vi "host.vi"() -> ()   [LabVIEW 2020]
uses:
  b4957acc-33c7-4f51-b6c8-be02e890b770.vi
  <vilib>/Array/Sort 2D Array - Pop Stack.vi
  <vilib>/Array/Sort 2D Array - Push Stack.vi
  b4957acc-33c7-4f51-b6c8-be02e890b770.vi/269d4b3b-47f5-49e3-8884-44851e4dd9d5.vi
  b4957acc-33c7-4f51-b6c8-be02e890b770.vi/6d99389c-673d-4efb-bf33-19b32bcf4cf8.vi
  <vilib>/FPGAPlugInAG/cRIO-9054/niLvFpga_Open_cRIO-9054.vi
  <vilib>/FPGAPlugInAG/cRIO-9054/niLvFpga_Reset_cRIO-9054.vi
  <vilib>/Utility/error.llb/Error Cluster From Error Code.vi
  <vilib>/rvi/errors/niLvFpgaAdjustHostInterfaceError.vi
  <vilib>/FPGAPlugInAG/cRIO-9054/niLvFpga_Run_cRIO-9054.vi
  <vilib>/FPGAPlugInAG/cRIO-9054/niLvFpga_Close_cRIO-9054.vi
  <vilib>/rvi/interface/nirviOpenFPGA/nirviOpenFPGA.xnode
  FPGA Bitfiles/latchproject_FPGATarget_FPGALatch2_iIOhPE-h5cE.lvbitx
  <vilib>/rvi/interface/nirviMethod/nirviMethod.xnode
  <vilib>/rvi/interface/nirviReadWriteControl/nirviReadWriteControl.xnode
  <vilib>/rvi/interface/nirviCloseFPGA/nirviCloseFPGA.xnode
  <vilib>/Analysis/NI_AALBase.lvlib
  <vilib>/rvi/errors/niLvFpgaMergeErrorWithErrorCode.vi
  <vilib>/FPGAPlugInAG/cRIO-9054/niLvFpga_StartFifo_cRIO-9054.vi
  <vilib>/FPGAPlugInAG/cRIO-9054/niLvFpga_ReadFifo_cRIO-9054.vi
  <vilib>/FPGAPlugInAG/cRIO-9054/niLvFpga_WriteFifo_cRIO-9054.vi
  NiFpgaLv.dll
panel:
  out "Timed Out? FIFO out index":bool
  out "Timed Out? FIFO out IMG":bool
  out "Timed Out? FIFO out REAL":bool
  out "Timed Out? FIFO in REAL":bool
  out "Timed Out? FIFO in IMG":bool
  out "sorted signal 3":dbl[](graph)
  out "Data":fxp<+/-,32,21>[](array[numeric])
  out "sorted signal 2":dbl[](graph)
  out "index values":i32[](array[numeric])
  out "sorted 2D array":dbl[][](array[numeric])
  out "appended array":dbl[][](array[numeric])
  out "sorted array":dbl[](array[numeric])
  out "uniform white noise":dbl[](array[numeric])
  out "Waveform Graph":sgl[](graph)
  out "sort time (ms)":dbl
  out "Elements Remaining":u32
  out "sorted signal":dbl[](graph)
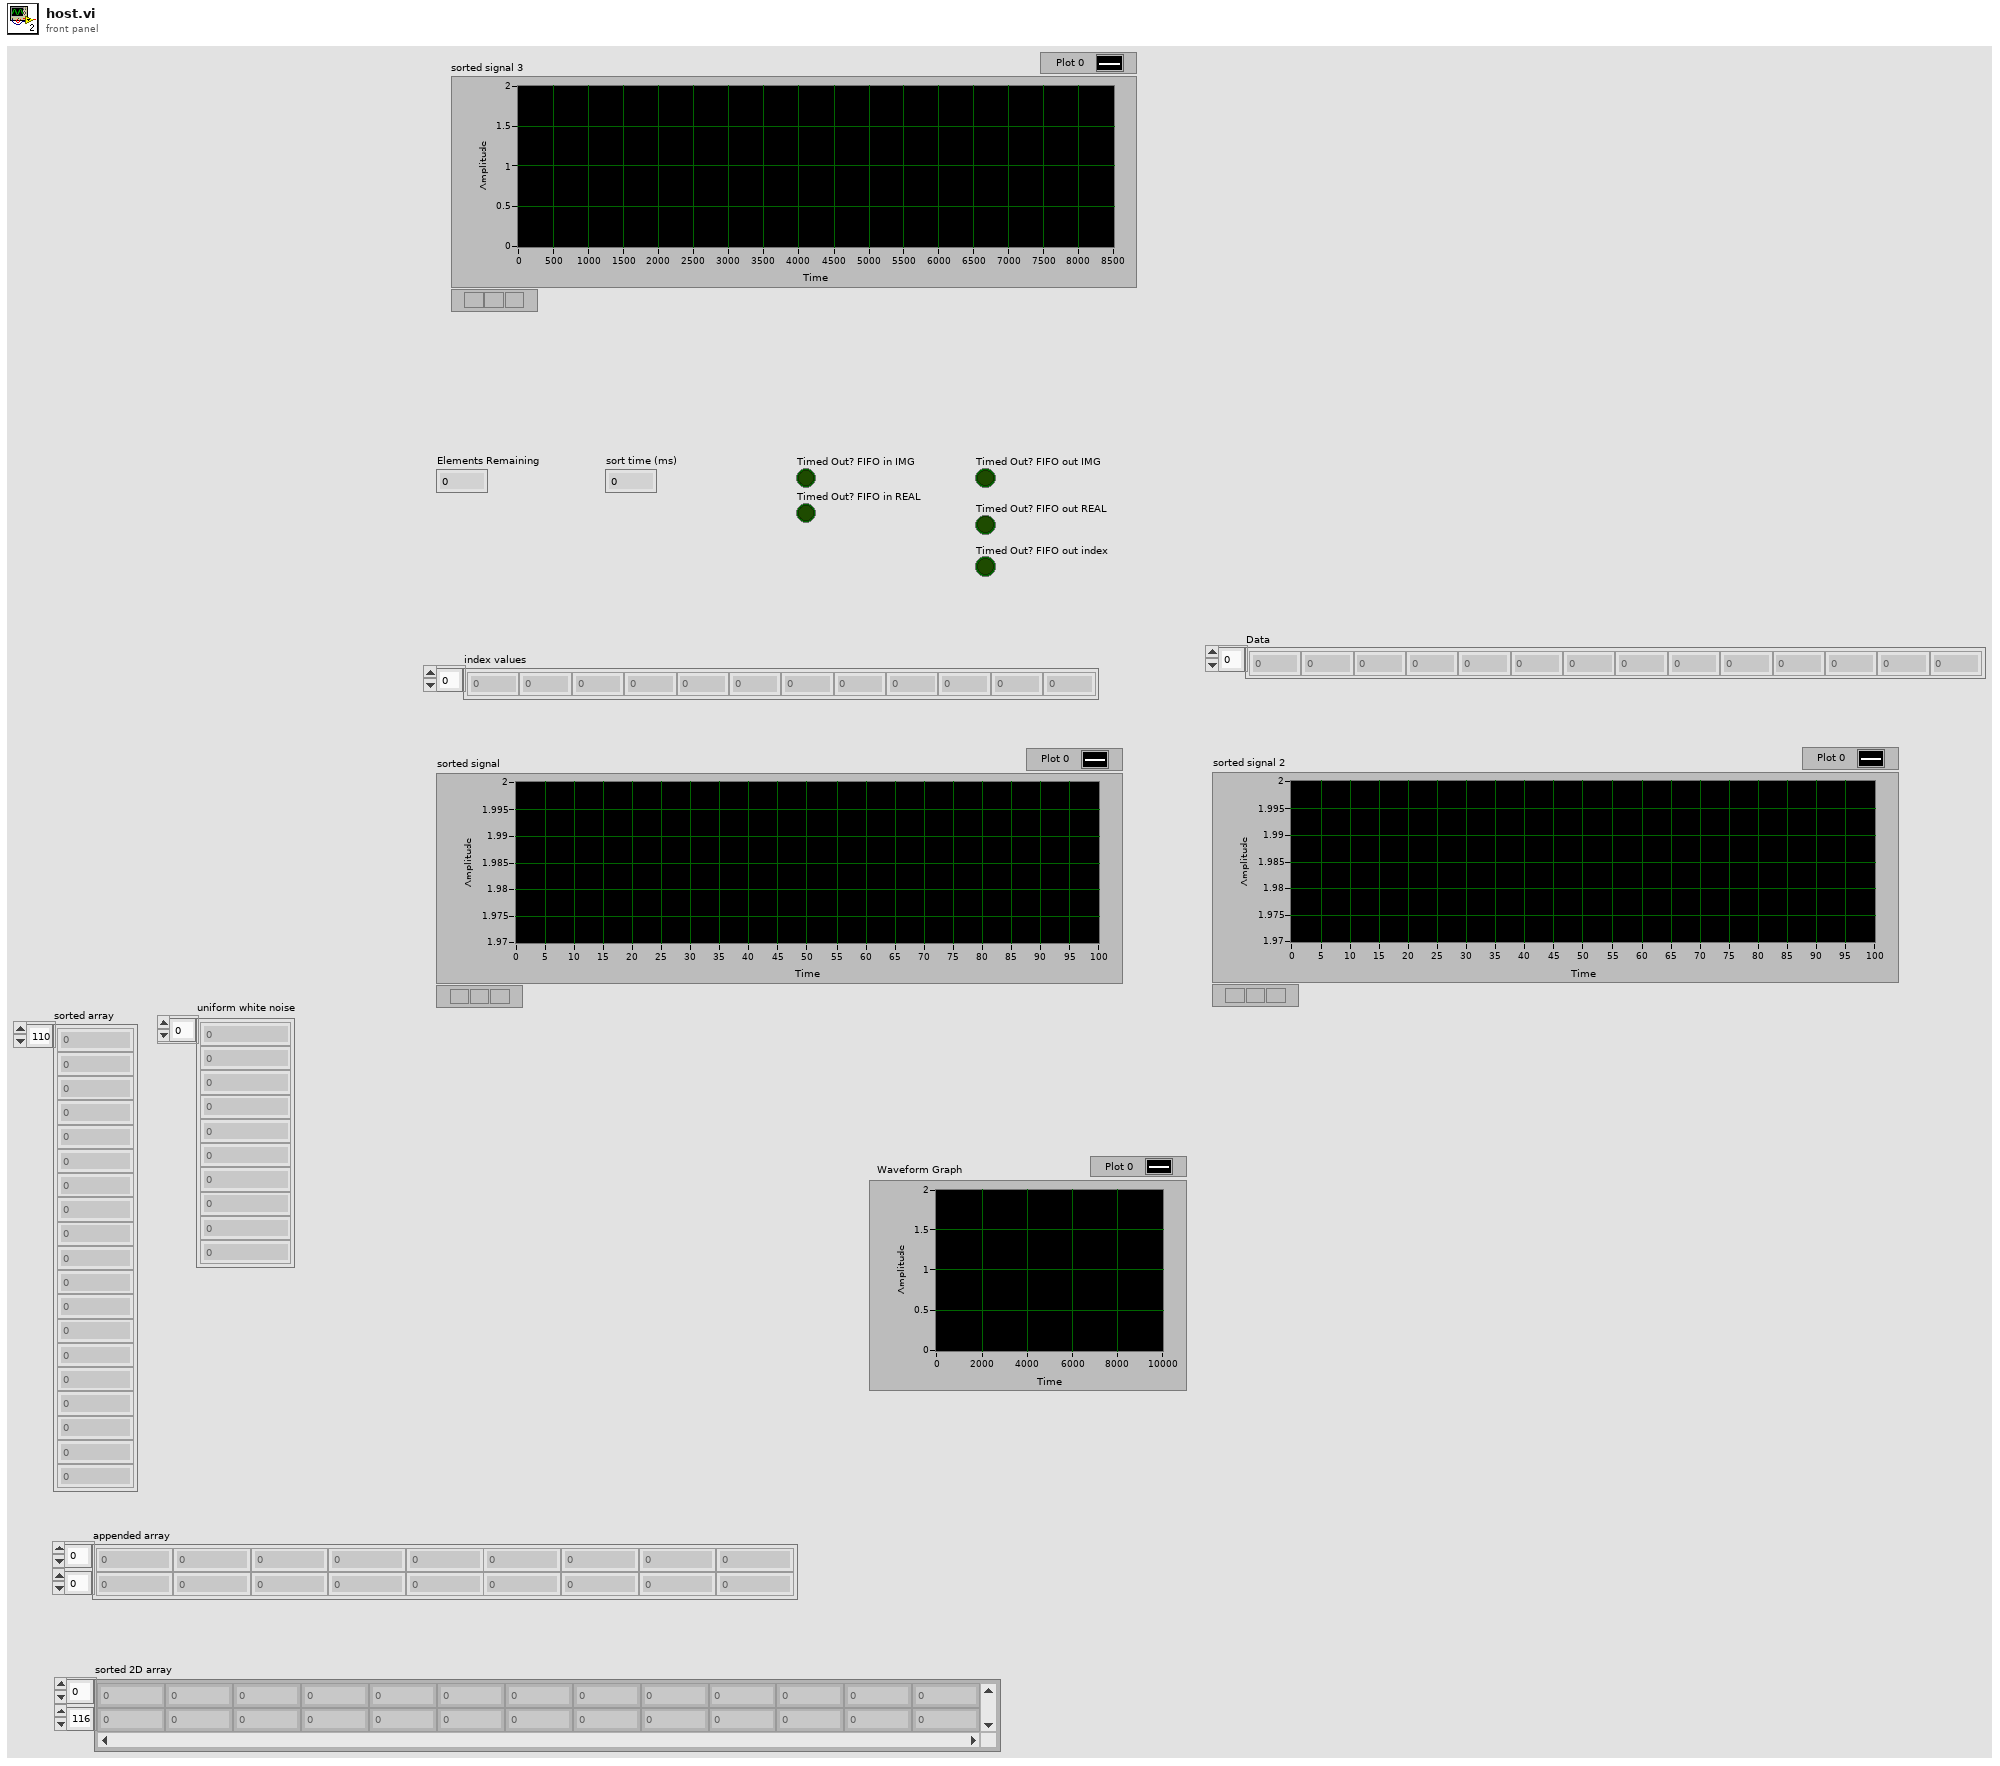
[diagram p1: front panel]
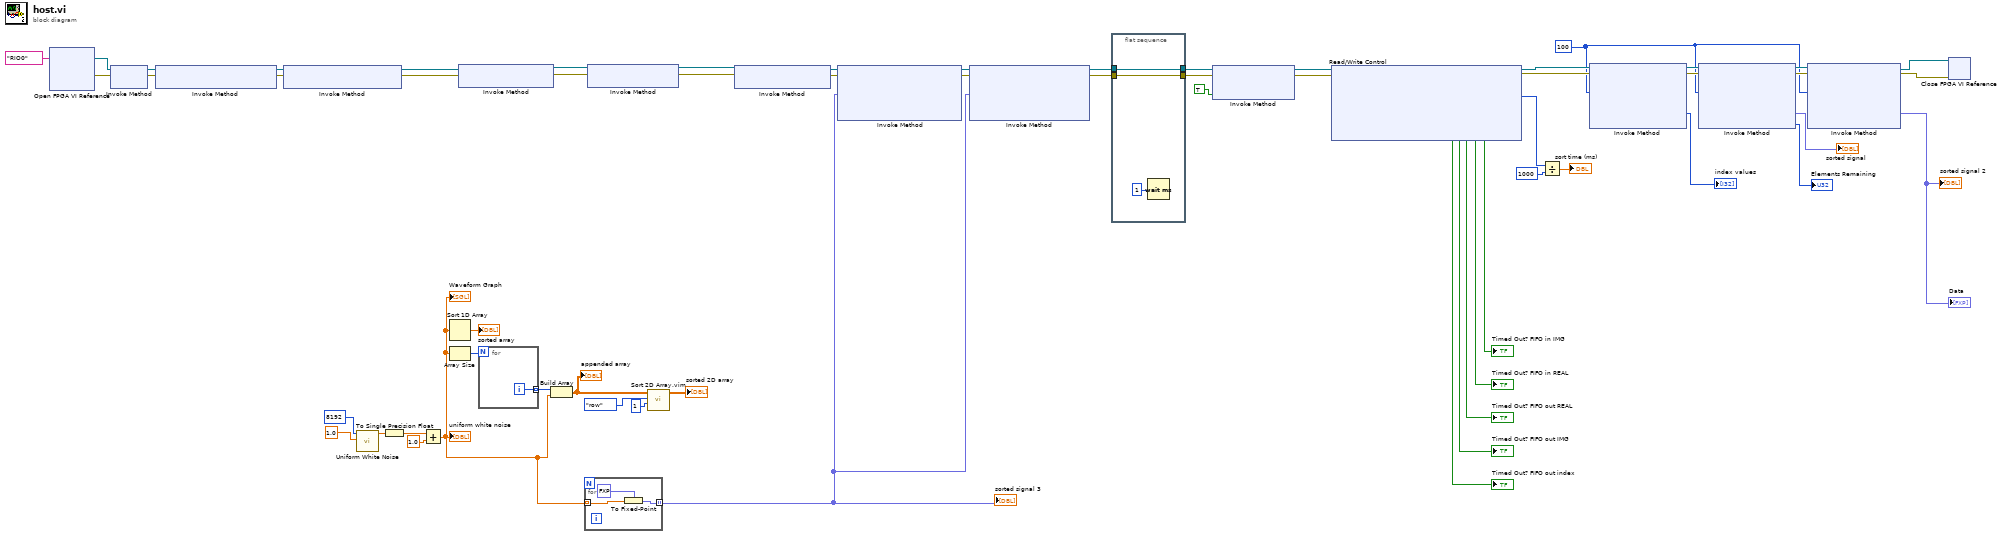
[diagram p0: block diagram]
diagram:
  w18 = u32 100 ("Number of Elements")
  n1 = xnode "Open FPGA VI Reference"("resource name"=tag "RIO0") -> ("FPGA VI Reference Out"=w57:refnum<k20>, "error out"=w56:errorcluster)  [unwired: 1 in]
  n2 = xnode "Invoke Method"("FPGA VI Reference In"=w57, "error in"=w56) -> ("FPGA VI Reference Out"=w59:refnum<k20>, "error out"=w58:errorcluster)
  n3 = xnode "Invoke Method"("FPGA VI Reference In"=w59, "error in"=w58) -> ("FPGA VI Reference Out"=w28:refnum<k20>, "error out"=w27:errorcluster)
  n4 = xnode "Invoke Method"("FPGA VI Reference In"=w28, "error in"=w27) -> ("FPGA VI Reference Out"=w13:refnum<k20>, "error out"=w12:errorcluster)
  n5 = call <vilib>:"Uniform White Noise.vi"("amplitude"=1.0, "samples"=8192) -> ("uniform white noise"=w31:dbl[])  [unwired: 8 in, 1 out]
  n6 = To Single Precision Float(number=w31) -> (single precision float=w30:sgl[])
  n7 = Add(x=w30, y=sgl 1.0 ("amplitude")) -> (x+y=w29:sgl[])
  "Waveform Graph" <- w29
  "uniform white noise" <- w29
  n8 = Sort 1D Array(array=w29) -> (sorted array=→"sorted array":sgl[])
  n9 = Array Size(array=w29) -> (size(s)=w38:i32)
  n10 = xnode "Invoke Method"("FPGA VI Reference In"=w13, "error in"=w12) -> ("FPGA VI Reference Out"=w11:refnum<k20>, "error out"=w16:errorcluster)
  n11 = for {
    N: w38 -> [_]
    tunnel: [w60] -> w37 mode=indexing
    i -> [w60]
  }
  n12 = Build Array(w37, w29) -> (w36:sgl[][])
  "appended array" <- w36
  n13 = for {
    tunnel: w29 -> [w63] mode=indexing
    tunnel: [w62] -> w10 mode=indexing
    n14 = To Fixed-Point(fixed-point type=fxp<+/-,32,21> 0.0, number=w63) -> (fixed-point=w62:fxp<+/-,32,21>)
  }
  "sorted signal 3" <- w10
  n15 = xnode "Invoke Method"("FPGA VI Reference In"=w11, "error in"=w16) -> ("FPGA VI Reference Out"=w15:refnum<k20>, "error out"=w14:errorcluster)
  n16 = call "Sort 2D Array.vim"("index"=1, "dimension to index (column)"=enum16{"column", "row"}."row", "2D array"=w36) -> ("sorted 2D array"=→"sorted 2D array":sgl[][])  [unwired: 7 in, 1 out]
  n17 = xnode "Invoke Method"("FPGA VI Reference In"=w15, "error in"=w14) -> ("FPGA VI Reference Out"=w26:refnum<k20>, "error out"=w25:errorcluster)
  n18 = xnode "Invoke Method"("FPGA VI Reference In"=w26, "error in"=w25, "Data"=w10) -> ("FPGA VI Reference Out"=w24:refnum<k20>, "error out"=w23:errorcluster)  [unwired: 1 in, 1 out]
  n19 = xnode "Invoke Method"("FPGA VI Reference In"=w24, "error in"=w23, "Data"=w10) -> ("FPGA VI Reference Out"=w3:refnum<k20>, "error out"=w1:errorcluster)  [unwired: 1 in, 1 out]
  n20 = flat-sequence {
    tunnel: [w65] -> w4
    tunnel: w3 -> [w65]
    tunnel: [w64] -> w2
    tunnel: w1 -> [w64]
    frame #0 {
      n21 = Wait (ms)(milliseconds to wait=u32 1) -> ()  [unwired: 1 out]
    }
  }
  n22 = xnode "Invoke Method"("FPGA VI Reference In"=w4, "error in"=w2, "Wait Until Done (F)"=TRUE) -> ("FPGA VI Reference Out"=w52:refnum<k20>, "error out"=w51:errorcluster)
  n23 = xnode "Read/Write Control"("FPGA VI Reference In"=w52, "error in"=w51) -> ("FPGA VI Reference Out"=w46:refnum<k20>, "error out"=w44:errorcluster, "sort time (us)"=w50:u32, "Timed Out? FIFO in IMG"=→"Timed Out? FIFO in IMG":bool, "Timed Out? FIFO in REAL"=→"Timed Out? FIFO in REAL":bool, "Timed Out? FIFO out REAL"=→"Timed Out? FIFO out REAL":bool, "Timed Out? FIFO out IMG"=→"Timed Out? FIFO out IMG":bool, "Timed Out? FIFO out index"=→"Timed Out? FIFO out index":bool)
  n24 = Divide(x=w50, y=u32 1000) -> (x/y=→"sort time (ms)":dbl)
  n25 = xnode "Invoke Method"("FPGA VI Reference In"=w46, "error in"=w44, "Number of Elements"=w18) -> ("FPGA VI Reference Out"=w45:refnum<k20>, "error out"=w43:errorcluster, "Data"=→"index values":i32[])  [unwired: 1 in, 1 out]
  n26 = xnode "Invoke Method"("FPGA VI Reference In"=w45, "error in"=w43, "Number of Elements"=w18) -> ("FPGA VI Reference Out"=w22:refnum<k20>, "error out"=w21:errorcluster, "Data"=→"sorted signal":fxp<+/-,32,21>[], "Elements Remaining"=→"Elements Remaining":u32)  [unwired: 1 in]
  n27 = xnode "Invoke Method"("FPGA VI Reference In"=w22, "error in"=w21, "Number of Elements"=w18) -> ("FPGA VI Reference Out"=w20:refnum<k20>, "error out"=w19:errorcluster, "Data"=→"sorted signal 2" →"Data":fxp<+/-,32,21>[])  [unwired: 1 in, 1 out]
  n28 = xnode "Close FPGA VI Reference"("FPGA VI Reference In"=w20, "error in"=w19) -> ()  [unwired: 1 out]
